vi "Change Voltage Channel 1.vi"(0 "object in":refnum<class "AFG3022B.lvclass">, 3 "Amplitude (1 Vpp)":dbl=1.0, 4 "Channel (0: Channel 1)":u16(ring)=1 items=["Channel 1", "Channel 2"], 5 "error in (no error)":errorcluster) -> (14 "object out":refnum<class "AFG3022B.lvclass">, 19 "error out":errorcluster)   [LabVIEW 2023, in "AFG3022B.lvclass"]
uses:
  AFG3022B.lvclass
  AFG3022B.lvclass/AFG3022B.ctl
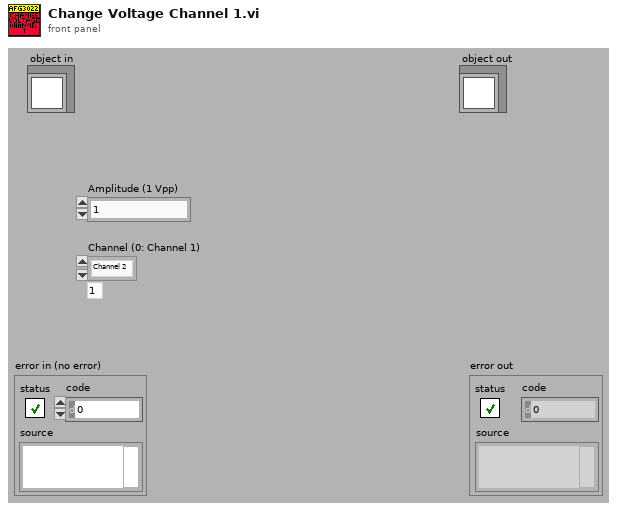
[diagram p1: front panel]
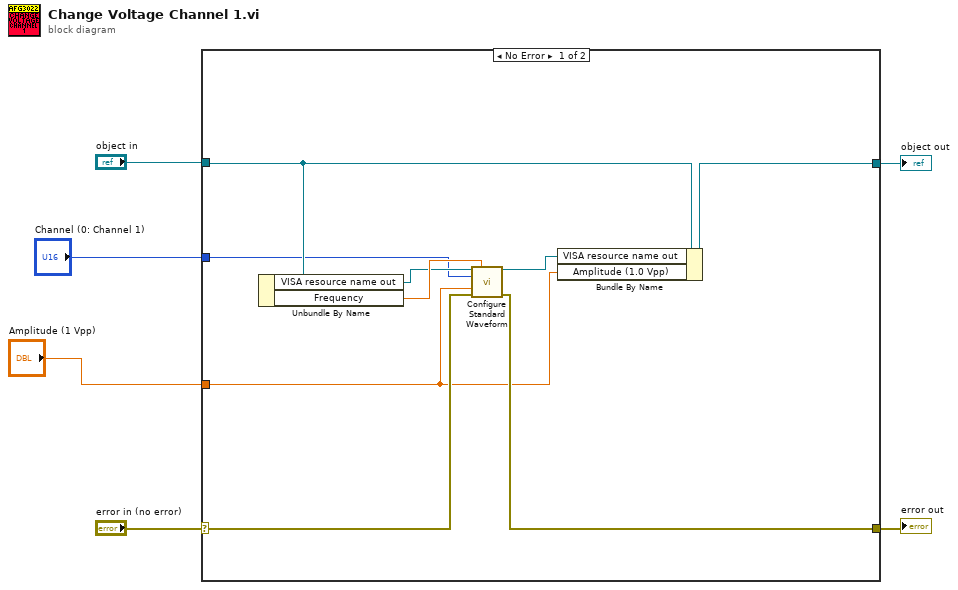
[diagram p0: block diagram]
diagram:
  n1 = case shown="No Error" "error in (no error)" {
    selector: "error in (no error)" -> [w9 w17]
    tunnel: [w8 w17] -> w5
    tunnel: [w14 w16] -> w3
    tunnel: "object in" -> [w15 w16]
    tunnel: "Channel (0: Channel 1)" -> [w10 _]
    tunnel: "Amplitude (1 Vpp)" -> [w7 _]
    frame No Error {
      n2 = Unbundle By Name(w15) -> ("VISA resource name out"=w12:refnum<visa-resource-name>, "Frequency"=w13:dbl)
      n3 = call <instrlib>:"Configure Standard Waveform.vi"("VISA resource name"=w12, "Frequency (1000 Hz)"=w13, "Channel (0: Channel 1)"=w10, "Amplitude (1 Vpp)"=w7, "error in (no error)"=w9) -> ("VISA resource name out"=w11:refnum<visa-resource-name>, "error out"=w8:errorcluster)  [unwired: 9 in]
      n4 = Bundle By Name(cluster=w15, "VISA resource name out"=w11, "Amplitude (1.0 Vpp)"=w7) -> (w14:refnum<class "AFG3022B.lvclass">)
    }
    frame Error {
    }
  }
  "error out" <- w5
  "object out" <- w3
